vi "FGV VI Ref Map.vi"(9 "Map Cmd":T1, 10 "VI Ref in":refnum<vi>, 11 "Class Name":string) -> (2 "VI Ref out":refnum<vi>, 3 "isExist":bool)   [LabVIEW 2023, in "Label-Driven UI.lvlib"]
uses:
  Label-Driven UI.lvlib
  Map Cmd.ctl
panel:
  out "Map":map{string, refnum<vi>}(c390)
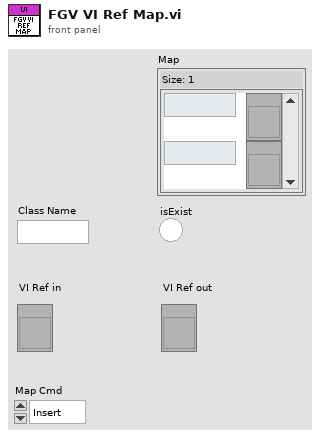
[diagram p1: front panel]
types:
  T1 = typedef "Label-Driven UI.lvlib/Map Cmd.ctl" = enum16{"Insert", "Delete", "Look"}
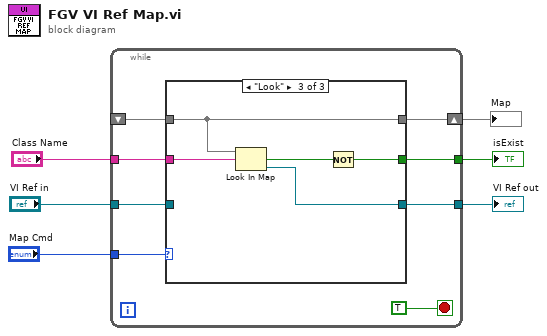
[diagram p0: block diagram]
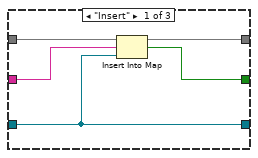
[diagram p2: hidden frame]
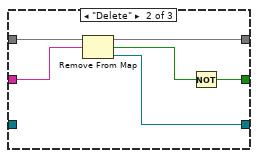
[diagram p3: hidden frame]
diagram:
  n1 = while {
    shift-right: [w14] -> w1
    shift-left: _ -> [w12]
    tunnel: "Map Cmd" -> [w13]
    tunnel: "Class Name" -> [w11]
    tunnel: "VI Ref in" -> [w10]
    tunnel: [w9] -> w4
    tunnel: [w8] -> w3
    stop <- TRUE stop-if-true
    n2 = case shown="\"Look\"" w13 {
      tunnel: [w18 w24 w30] -> w14
      tunnel: w12 -> [w19 w25 w30]
      tunnel: w11 -> [w17 w23 w29]
      tunnel: w10 -> [w15 _ _]
      tunnel: [w16 w20 w26] -> w9
      tunnel: [w15 w21 w27] -> w8
      frame "Insert" {
        n3 = Insert Into Map(map in=w19, key=w17, value=w15) -> (map out=w18:map{string, refnum<vi>}, key already included?=w16:bool)  [unwired: 1 out]
      }
      frame "Delete" {
        n4 = Remove From Map(10:w23, 11:w25) -> (1:w21:refnum<vi>, 2:w22:bool, 3:w24:map{string, refnum<vi>})
        n5 = Not(x=w22) -> (.not. x?=w20:bool)
      }
      frame "Look" {
        n6 = Look In Map(map=w30, key=w29) -> (key not found?=w28:bool, value=w27:refnum<vi>)  [unwired: 1 in]
        n7 = Not(x=w28) -> (.not. x?=w26:bool)
      }
    }
  }
  "isExist" <- w4
  "VI Ref out" <- w3
  "Map" <- w1
